vi "On.vi"(8 "error in (no error)":errorcluster, 11 "ThAr in":refnum<class "ThAr.lvclass">) -> (0 "error out":errorcluster, 3 "ThAr out":refnum<class "ThAr.lvclass">)   [LabVIEW 2016, in "ThAr.lvclass"]
uses:
  ThAr.lvclass
  Lamp.lvclass
panel:
  out "Bytes Written":u32
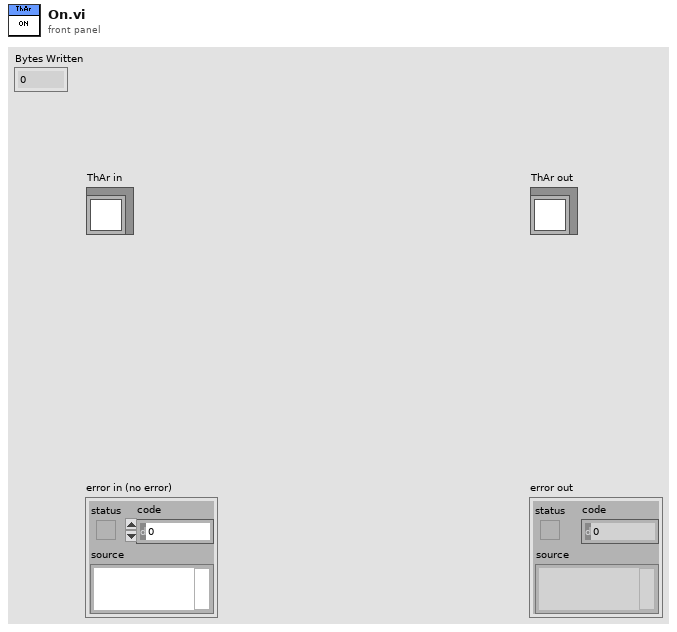
[diagram p1: front panel]
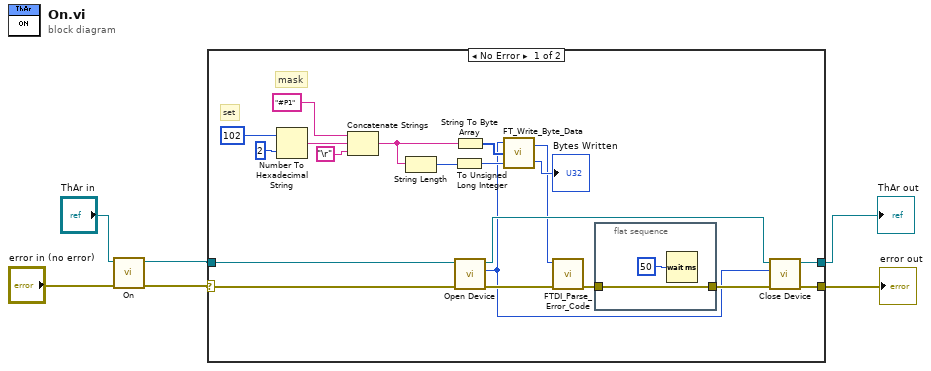
[diagram p0: block diagram]
diagram:
  n1 = call-parent "On.vi"("error in (no error)"="error in (no error)", "Lamp in"="ThAr in") -> ("error out"=w3:errorcluster, "Lamp out"=w4:refnum<class "ThAr.lvclass">)  [unwired: 8 in]
  n2 = case shown="No Error" w3 {
    selector: w3 -> [w12 w30]
    tunnel: [w18 w30] -> w1
    tunnel: w4 -> [w11 w29]
    tunnel: [w8 w29] -> w2
    frame No Error {
      # "set"
      # "mask"
      n3 = Number To Hexadecimal String(1:i16 2 ("width (-)"), 2:102 ("number")) -> (0:w25:string)
      n4 = Concatenate Strings("#P1" ("Substring"), w25, "\r") -> (w19:string)
      n5 = String Length(string=w19) -> (length=w23:i32)
      n6 = To Unsigned Long Integer(number=w23) -> (unsigned 32bit integer=w22:u32)
      n7 = String To Byte Array(string=w19) -> (unsigned byte array=w21:u8[])
      n8 = call "Open Device.vi"("error in (no error)"=w12, "ThAr in"=w11) -> ("error constant"=w17:errorcluster, "Handle"=w7:u32, "ThAr out"=w10:refnum<class "ThAr.lvclass">)  [unwired: 7 in]
      n9 = call "FT_Write_Byte_Data.vi"("Bytes To Write"=w22, "Buffer"=w21, "Handle"=w7) -> ("Bytes Written"=→"Bytes Written":u32, "FT_Status"=w9:u32)
      n10 = call "FTDI_Parse_Error_Code.vi"("error in (no error)"=w17, "FT_Status"=w9) -> ("error out"=w16:errorcluster)  [unwired: 9 in]
      n11 = flat-sequence {
        tunnel: w16 -> [w27]
        tunnel: [w27] -> w15
        frame #0 {
          n12 = Wait (ms)(milliseconds to wait=u32 50) -> ()  [unwired: 1 out]
        }
      }
      n13 = call "Close Device.vi"("error in (no error)"=w15, "Handle"=w7, "ThAr in"=w10) -> ("error out"=w18:errorcluster, "ThAr out"=w8:refnum<class "ThAr.lvclass">)  [unwired: 7 in]
    }
    frame Error {
    }
  }
  "error out" <- w1
  "ThAr out" <- w2
